vi "Load Settings from File.vi"(8 "error in":errorcluster) -> (0 "error out":errorcluster, 2 "Dashboard Data (out)":T1={"Drive PID - Low"={"D"=0.0, "F"=0.0, "RR"=0.0, "IZ"=0.0, "P"=0.0, "I"=0.0}, "Drive PID - High"={"D"=0.0, "F"=0.0, "RR"=0.0, "IZ"=0.0, "P"=0.0, "I"=0.0}, "Vision Settings"={"LED Color"={"Hue"={107.81818389892578, 139.81818389892578}, "Sat"={176.07142857142858, 255.0}, "Val"={40.53571428571429, 255.0}}, "Vision Line"=0.0}, "Robot Name"="", "Winch Out"=0.0, "Winch In"=0.0, "Shooter Settings"={"Shooter PID"={"D"=0.0, "F"=0.0, "RR"=0.0, "IZ"=0.0, "P"=0.0, "I"=0.0}, "Instake Belt PID"={"D"=0.0, "F"=0.0, "RR"=0.0, "IZ"=0.0, "P"=0.0, "I"=0.0}, "Shooter Wheel RPM"=0.0, "Instake Belt RPM"=0.0, "Grinder Power"=0.0, "Ramp Up Speed"=0.0}, "Auto Start"=enum."Left"} {"Vision Settings"."LED Color"."Hue" scale=0.0..255.0 scale format="%#_3g"}, 3 "refnum out":T6)   [LabVIEW 2016]
uses:
  <vilib>/Utility/config.llb/NI_LVConfig.lvlib
  <vilib>/Utility/config.llb/Config Data RefNum.ctl
  Load Save Info.ctl
  PID Settings.ctl
  Dashboard Data.ctl
  Shooter Settings.ctl
  AutoPositions Type Def.ctl
  Vision Data.ctl
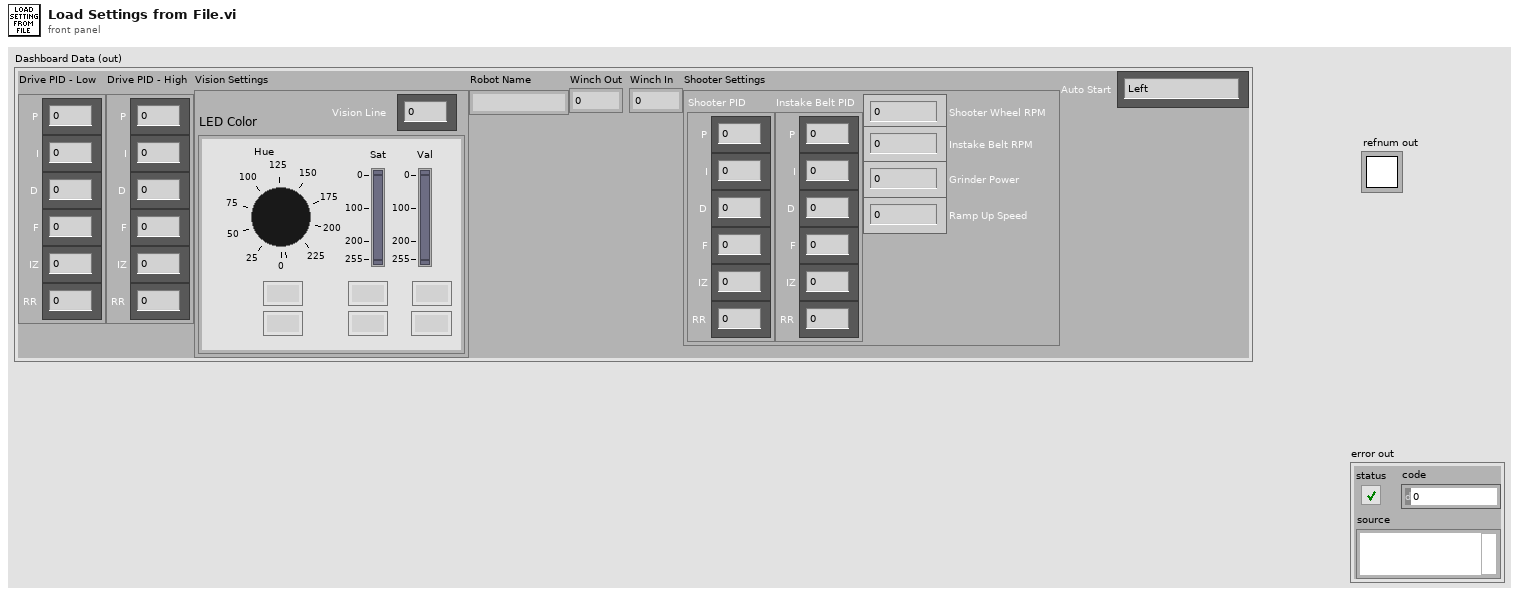
[diagram p1: front panel]
types:
  T1 = typedef "Dashboard Data.ctl" = cluster{"Drive PID - Low":T2, "Drive PID - High":T2, "Vision Settings":T3, "Robot Name":string, "Winch Out":dbl, "Winch In":dbl, "Shooter Settings":T4, "Auto Start":T5}
  T2 = typedef "PID Settings.ctl" = cluster{"D":dbl, "F":dbl, "RR":dbl, "IZ":dbl, "P":dbl, "I":dbl}
  T3 = typedef "Vision Data.ctl" = cluster{"LED Color":cluster{"Hue":cluster{dbl, dbl}, "Sat":cluster{dbl, dbl}, "Val":cluster{dbl, dbl}}, "Vision Line":dbl}
  T4 = typedef "Shooter Settings.ctl" = cluster{"Shooter PID":T2, "Instake Belt PID":T2, "Shooter Wheel RPM":dbl, "Instake Belt RPM":dbl, "Grinder Power":dbl, "Ramp Up Speed":dbl}
  T5 = typedef "AutoPositions Type Def.ctl" = enum16{"Left", "Middle", "Right"}
  T6 = typedef "NI_LVConfig.lvlib/Config Data RefNum.ctl" = refnum<k1>
  T7 = typedef "Load Save Info.ctl" = cluster{"Load?":bool, "Dashboard?":bool, "save file":T6, "File?":bool}
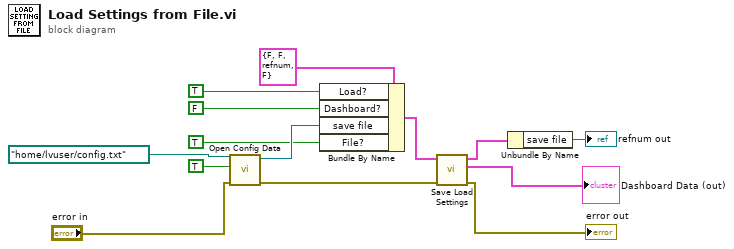
[diagram p0: block diagram]
diagram:
  n1 = call <vilib>:"Open Config Data.vi"("error in (no error)"="error in", "create file if necessary (T)"=TRUE, "configuration file path"=path "/home/lvuser/config.txt" ("file path (use dialog)")) -> ("error out"=w10:errorcluster, "refnum"=w5:T6)  [unwired: 6 in, 1 out]
  n2 = Bundle By Name(cluster=T7 {"Load?"=FALSE, "Dashboard?"=FALSE, "save file"=refnum, "File?"=FALSE} ("Save Load Info"), "Load?"=TRUE, "Dashboard?"=FALSE, "save file"=w5, "File?"=TRUE) -> (w8:T7)
  n3 = call "Save Load Settings.vi"("error in"=w10, "Save Load Info"=w8) -> ("error out"=→"error out":errorcluster, "Dashboard Data (out)"=→"Dashboard Data (out)":T1, "Save Load Info (out)"=w3:T7)  [unwired: 7 in]
  n4 = Unbundle By Name(w3) -> ("save file"=→"refnum out":T6)
